vi "Voronoi_Voronoi Edges.vi"(10 "Y":dbl[](array[numeric]), 11 "X":dbl[](array[numeric])) -> (0 "error":i32, 2 "Edge Y":dbl[][](array[numeric]), 3 "Edge X":dbl[][](array[numeric]))   [LabVIEW 2017, in "NI_AAL_Geometry.lvlib"]
uses:
  <vilib>/Analysis/NI_AAL_Geometry.lvlib
  <vilib>/Analysis/geometry.llb/DT_Output Option.ctl
panel:
  # "Voronoi Edges"
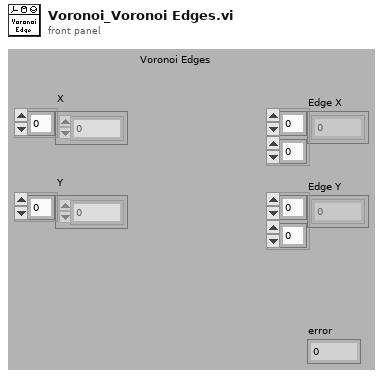
[diagram p1: front panel]
types:
  T1 = typedef "NI_AAL_Geometry.lvlib/DT_Output Option.ctl" = i32
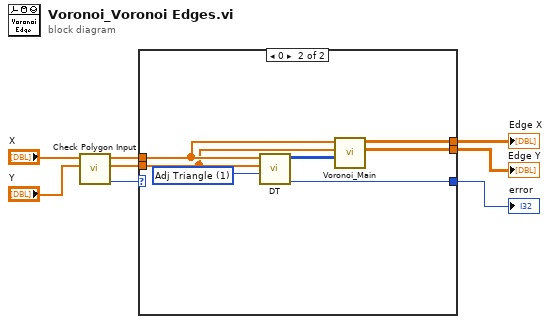
[diagram p0: block diagram]
diagram:
  n1 = call <vilib>:"Check Polygon Input.vi"("Y In"="Y", "X In"="X") -> ("error"=w5:i32, "Y Out"=w1:dbl[], "X Out"=w2:dbl[])  [unwired: 7 in]
  n2 = case shown="0" w5 {
    selector: w5 -> [w9 _]
    tunnel: [w9 w11] -> w6
    tunnel: [_ w15] -> w8
    tunnel: [_ w14] -> w7
    tunnel: w2 -> [_ w13]
    tunnel: w1 -> [_ w12]
    frame -1, Default {
    }
    frame 0 {
      w10 = T1 1 items=["Triangle", "Adj Triangle", "Segment"] ("output option")
      n3 = call <vilib>:"DT.vi"("output option"=w10, "Y"=w12, "X"=w13) -> ("error"=w11:i32, "Triangles"=w16:i32[][])  [unwired: 7 in]
      n4 = call <vilib>:"Voronoi_Main.vi"("Triangles"=w16, "Y"=w12, "X"=w13) -> ("Edge Y"=w14:dbl[][], "Edge X"=w15:dbl[][])  [unwired: 7 in]
    }
  }
  "Edge X" <- w8
  "Edge Y" <- w7
  "error" <- w6
